vi "ResetArmSoftlimits.vi"   [LabVIEW 2015]
uses:
  Framework/Motor Ref Names Type Def.ctl
  Framework/Robot Global Data.vi
types:
  T1 = typedef "Motor Ref Names Type Def.ctl" = enum16{"Angular Motor", "Shooter Motor Bottom", "Shooter Motor Top", "Arm Shooter Motor"}
  T2 = typedef "Addon Motor Type Def.ctl" = cluster{"SwitchDevRef":T3, "LidarRef":T6, "Arm Sensors":cluster{"Front Sensor":T3, "Back Sensor":T3, "Ball Sensor":T3}}
  T3 = typedef "WPI_SwitchDevRef.ctl" = cluster{"DevStatus":errorcluster, "DIO Channel":T4, "CntIndex":T5, "Normally Closed":bool}
  T4 = typedef "FPGA_DIOChannel.ctl" = enum8{"DIO 0", "DIO 1", "DIO 2", "DIO 3", "DIO 4", "DIO 5", "DIO 6", "DIO 7", "DIO 8", "DIO 9", "DIO MXP 0", "DIO MXP 1", "DIO MXP 2", "DIO MXP 3", "DIO MXP 4", "DIO MXP 5", "DIO MXP 6", "DIO MXP 7", "DIO MXP 8", "DIO MXP 9", "DIO MXP 10", "DIO MXP 11", "DIO MXP 12", "DIO MXP 13", "DIO MXP 14", "DIO MXP 15", "Invalid"}
  T5 = typedef "FPGA_CounterCtrSystemIndex.ctl" = enum8{"Ctr 0", "Ctr 1", "Ctr 2", "Ctr 3", "Ctr 4", "Ctr 5", "Ctr 6", "Ctr 7", "Invalid"}
  T6 = typedef "Lidar Type Def.ctl" = cluster{"I2CDevRef":T7}
  T7 = typedef "WPI_I2CDevRef.ctl" = cluster{"DevStatus":errorcluster, "Device Address":u8, "Handle":i32, "I2C Bus":T8}
  T8 = typedef "i2c_bus.ctl" = enum16{"I2C On-Board", "I2C MXP", "Invalid"}
  T9 = typedef "Motor Ref Array Type Def.ctl" = T10[]
  T10 = typedef "Detailed Motor Type Def.ctl" = cluster{"MotorRef":T11, "Encoder Ticks Per Rev":dbl, "Set Position":dbl}
  T11 = typedef "WPI_MotorControlDeviceRef.ctl" = cluster{"DeviceStatus":errorcluster, "Type":T12, "PWM":cluster{"PWM Channel":T13, "DeadBand":T14}, "CAN":cluster{"Device Number":u8, "Control Mode":T15, "Semaphore":T16, "Max Vout":dbl, "TalonSRX Control Mode":T17}, "Invert":bool}
  T12 = typedef "WPI_MotorControlType.ctl" = enum16{"PWM", "CAN", "CANTalonSRX"}
  T13 = typedef "FPGA_DIOPWMChannel.ctl" = enum8{"PWM 0", "PWM 1", "PWM 2", "PWM 3", "PWM 4", "PWM 5", "PWM 6", "PWM 7", "PWM 8", "PWM 9", "PWM MXP 0", "PWM MXP 1", "PWM MXP 2", "PWM MXP 3", "PWM MXP 4", "PWM MXP 5", "PWM MXP 6", "PWM MXP 7", "PWM MXP 8", "PWM MXP 9", "Invalid"}
  T14 = typedef "WPI_PWMDeadband.ctl" = cluster{"Name":string, "maxPositivePwm":i32, "minPositivePwm":i32, "centerPwm":i32, "maxNegativePwm":i32, "minNegativePwm":i32, "angularRange":u16}
  T15 = typedef "WPI_CANJaguar_ControlMode.ctl" = enum8{"Percent VBus", "Current", "Speed", "Position", "Voltage"}
  T16 = typedef "Semaphore RefNum" = refnum<k1>
  T17 = typedef "WPI_CANTalonSRX_APIControlMode.ctl" = enum8{"Percent VBus", "Speed", "Position", "Slave", "Unchanged / Invalid", "Voltage Compensation", "Current", "Motion Profile"}
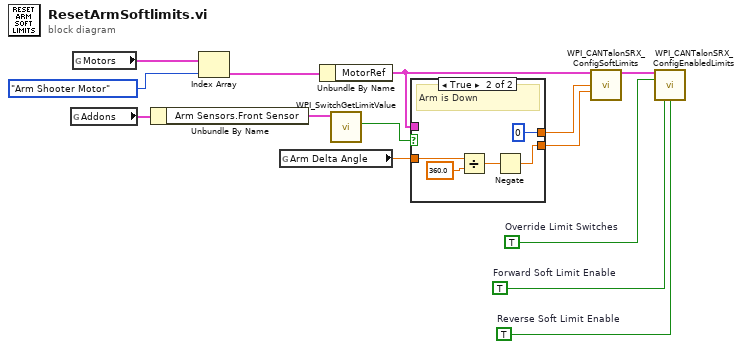
[diagram p0: block diagram]
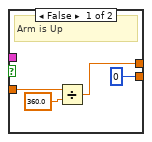
[diagram p2: hidden frame]
diagram:
  w1 = TRUE  # Reverse Soft Limit Enable
  w2 = TRUE  # Forward Soft Limit Enable
  w3 = TRUE  # Override Limit Switches
  n1 = global read "Robot Global Data.vi" "Addons"() -> (w11:T2)
  n2 = global read "Robot Global Data.vi" "Motors"() -> (w14:T9)
  n3 = Unbundle By Name(w11) -> ("Arm Sensors.Front Sensor"=w10:T3)
  n4 = Index Array(array=w14, index=Motor_Ref_Names_Type_Def."Arm Shooter Motor" ("Motor Ref Names")) -> (element=w12:T10)
  n5 = global read "Robot Global Data.vi" "Arm Delta Angle"() -> (w6:dbl)
  n6 = Unbundle By Name(w12) -> ("MotorRef"=w8:T11)
  n7 = call <vilib>:"WPI_SwitchGetLimitValue.vi"("SwitchDevRef"=w10) -> ("Switch Pressed"=w9:bool)  [unwired: 8 in, 2 out]
  n8 = case shown="True" w9 {
    tunnel: w8 -> [_ _]
    tunnel: [w15 0] -> w7
    tunnel: w6 -> [w16 w22]
    tunnel: [0 w20] -> w5
    frame False {
      # "Arm is Up"
      n9 = Divide(x=w16, y=360.0) -> (x/y=w15:dbl)
    }
    frame True {
      # "Arm is Down"
      n10 = Divide(x=w22, y=360.0) -> (x/y=w19:dbl)
      n11 = Negate(x=w19) -> (-x=w20:dbl)
    }
  }
  n12 = call <vilib>:"WPI_CANTalonSRX_ConfigSoftLimits.vi"("CAN Talon SRX Ref"=w8, "Forward Limit Position"=w7, "Reverse Limit Position"=w5) -> ("CAN Talon SRX Ref"=w4:T11)  [unwired: 11 in, 1 out]
  n13 = call <vilib>:"WPI_CANTalonSRX_ConfigEnabledLimits.vi"("CAN Talon SRX Ref"=w4, "Override Limit Switches"=w3, "Forward Soft Limit Enable"=w2, "Reverse Soft Limit Enable"=w1) -> ()  [unwired: 10 in, 2 out]
